vi "Register for Actor Stop Event.vi"(8 "error in (no error)":errorcluster, 9 "Event Registration Refnum in":refnum<event-registration>, 11 "CO2 Actor in":refnum<class "CO2 Actor.lvclass">) -> (0 "error out":errorcluster, 1 "Event Registration Refnum":refnum<event-registration>, 3 "CO2 Actor out":refnum<class "CO2 Actor.lvclass">)   [LabVIEW 2015, in "cRIO-Carbondioxide.lvlib" / "CO2-Actor.lvlib" / "CO2 Actor.lvclass"]
uses:
  CO2 Actor.lvclass
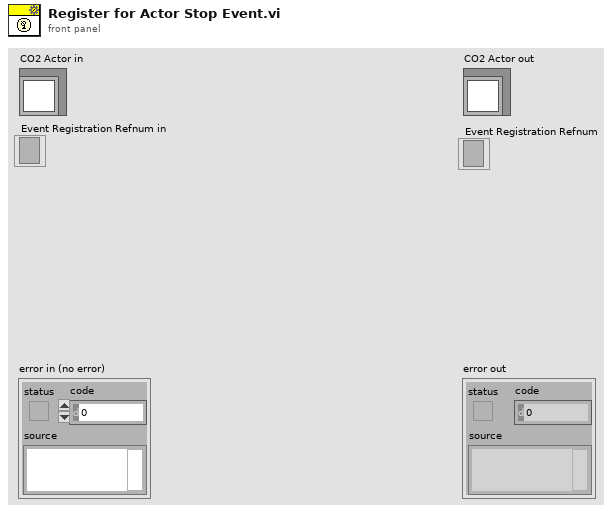
[diagram p1: front panel]
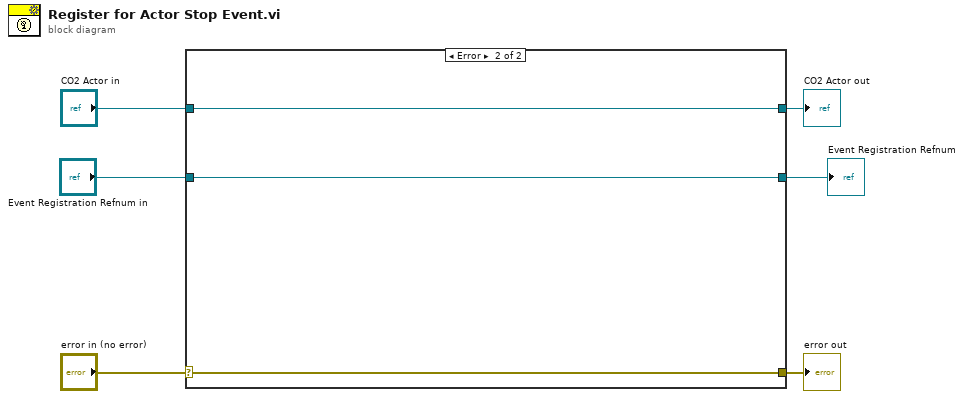
[diagram p0: block diagram]
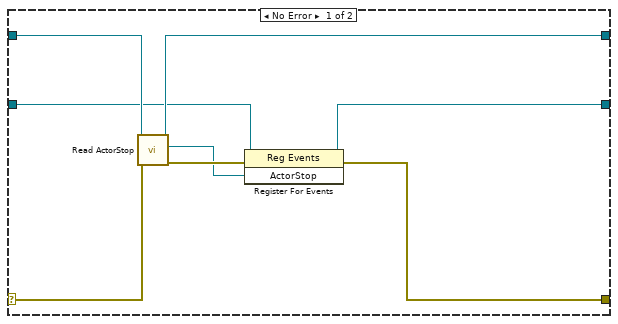
[diagram p2: hidden frame]
diagram:
  n1 = case shown="Error" "error in (no error)" {
    selector: "error in (no error)" -> [w8 w17]
    tunnel: [w7 w17] -> w5
    tunnel: [w11 w16] -> w3
    tunnel: "CO2 Actor in" -> [w12 w16]
    tunnel: [w9 w15] -> w2
    tunnel: "Event Registration Refnum in" -> [w10 w15]
    frame No Error {
      n2 = call "Read ActorStop.vi"("error in (no error)"=w8, "CO2 Actor in"=w12) -> ("error out"=w14:errorcluster, "ActorStop"=w13:refnum<user-event>, "CO2 Actor out"=w11:refnum<class "CO2 Actor.lvclass">)  [unwired: 7 in]
      n3 = register-events(reference=w10, error in=w14, w13) -> (reference out=w9:refnum<event-registration>, error out=w7:errorcluster)
    }
    frame Error {
    }
  }
  "error out" <- w5
  "CO2 Actor out" <- w3
  "Event Registration Refnum" <- w2
